vi "Decode Inverter Command Modes.vi"(11 "Numeric":u8) -> (3 "Inv. Command":enum16{"CAN Mode", "VSM Mode"}(ring))   [LabVIEW 2015]
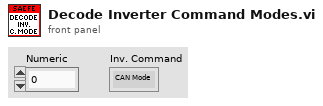
[diagram p1: front panel]
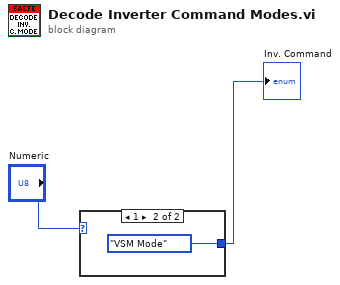
[diagram p0: block diagram]
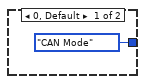
[diagram p2: hidden frame]
diagram:
  n1 = case shown="1" "Numeric" {
    tunnel: [enum16{"CAN Mode", "VSM Mode"}."CAN Mode" ("Inv. Command") enum16{"CAN Mode", "VSM Mode"}."VSM Mode" ("Inv. Command")] -> w2
    frame 0, Default {
    }
    frame 1 {
    }
  }
  "Inv. Command" <- w2
